vi "Get Neighbor Coordinates.vi"(8 "# cols":i32, 9 "# rows":i32, 10 "column":i32, 11 "row":i32) -> (3 "neighbor coordinates":i32[][](array[numeric]))   [LabVIEW 2021, in "Game of Life.lvlib"]
doc: "This VI gets the coordinates of the neighboring cells."
uses:
  Game of Life.lvlib
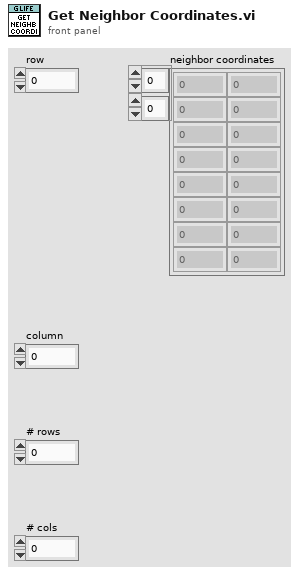
[diagram p1: front panel]
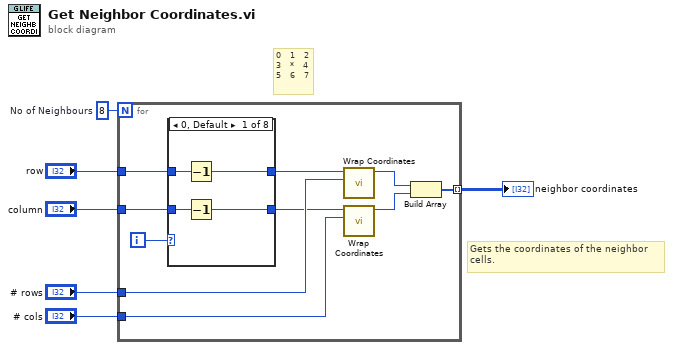
[diagram p0: block diagram]
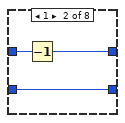
[diagram p2: hidden frame]
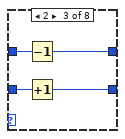
[diagram p3: hidden frame]
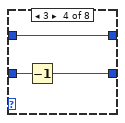
[diagram p4: hidden frame]
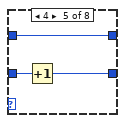
[diagram p5: hidden frame]
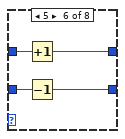
[diagram p6: hidden frame]
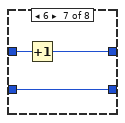
[diagram p7: hidden frame]
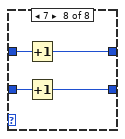
[diagram p8: hidden frame]
diagram:
  w1 = 8  # No of Neighbours
  # "Gets the coordinates of the neighbor\ncells."
  # "0   1   2\n3   *   4\n5   6   7"
  n1 = for {
    N: w1 -> [_]
    tunnel: "row" -> [w15]
    tunnel: "column" -> [w14]
    tunnel: [w13] -> w2 mode=indexing
    tunnel: "# rows" -> [w11]
    tunnel: "# cols" -> [w8]
    i -> [w16]
    n2 = case shown="0, Default" w16 {
      tunnel: w15 -> [w20 w23 w27 w28 w31 w37 w40 w44]
      tunnel: w14 -> [w19 w21 w26 w30 w33 w36 w38 w43]
      tunnel: [w18 w22 w25 w28 w31 w35 w39 w42] -> w12
      tunnel: [w17 w21 w24 w29 w32 w34 w38 w41] -> w9
      frame 0, Default {
        n3 = Decrement(x=w20) -> (x-1=w18:i32)
        n4 = Decrement(x=w19) -> (x-1=w17:i32)
      }
      frame 1 {
        n5 = Decrement(x=w23) -> (x-1=w22:i32)
      }
      frame 2 {
        n6 = Decrement(x=w27) -> (x-1=w25:i32)
        n7 = Increment(x=w26) -> (x+1=w24:i32)
      }
      frame 3 {
        n8 = Decrement(x=w30) -> (x-1=w29:i32)
      }
      frame 4 {
        n9 = Increment(x=w33) -> (x+1=w32:i32)
      }
      frame 5 {
        n10 = Increment(x=w37) -> (x+1=w35:i32)
        n11 = Decrement(x=w36) -> (x-1=w34:i32)
      }
      frame 6 {
        n12 = Increment(x=w40) -> (x+1=w39:i32)
      }
      frame 7 {
        n13 = Increment(x=w44) -> (x+1=w42:i32)
        n14 = Increment(x=w43) -> (x+1=w41:i32)
      }
    }
    n15 = call "Wrap Coordinates.vi"("length"=w11, "index"=w12) -> ("translated index"=w10:i32)  [unwired: 9 in]
    n16 = call "Wrap Coordinates.vi"("length"=w8, "index"=w9) -> ("translated index"=w7:i32)  [unwired: 9 in]
    n17 = Build Array(w10, w7) -> (w13:i32[])
  }
  "neighbor coordinates" <- w2
